vi "Initialize.vi"(8 "error in (no error)":errorcluster, 11 "reference in":refnum<class "Timing.lvclass">) -> (0 "error out":errorcluster, 3 "reference out":refnum<class "Timing.lvclass">)   [LabVIEW 2019, in "Timing.lvclass"]
doc: "Initializes module"
uses:
  Timing.lvclass
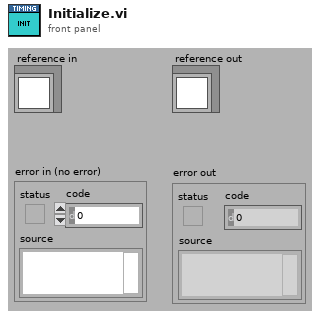
[diagram p1: front panel]
types:
  T1 = typedef "Timing.lvclass/ObjectAttributes.ctl" = cluster{"MyAttribute":dbl}
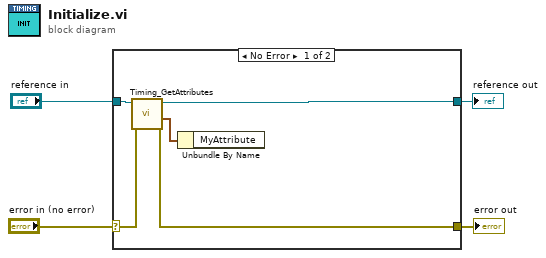
[diagram p0: block diagram]
diagram:
  n1 = case shown="No Error" "error in (no error)" {
    selector: "error in (no error)" -> [w9 w11]
    tunnel: [w8 w11] -> w3
    tunnel: [w7 w10] -> w1
    tunnel: "reference in" -> [w5 w10]
    frame No Error {
      n2 = call "Timing_GetAttributes.vi"("error in (no error)"=w9, "reference in"=w5) -> ("error out"=w8:errorcluster, "attributes"=w6:T1, "reference out"=w7:refnum<class "Timing.lvclass">)  [unwired: 6 in, 1 out]
      n3 = Unbundle By Name(w6) -> ()  [unwired: 1 out]
    }
    frame Error {
    }
  }
  "error out" <- w3
  "reference out" <- w1
